vi "AOL Z Cal-Ctrl visibility.vi"(8 "error in (no error)":errorcluster, 11 "State":T1=enum."Select cal mode") -> (0 "error out":errorcluster)   [LabVIEW 2020]
uses:
  Typedefs/AOL Z cal wizard states.ctl
  Globals/gl_Calibration globals.vi
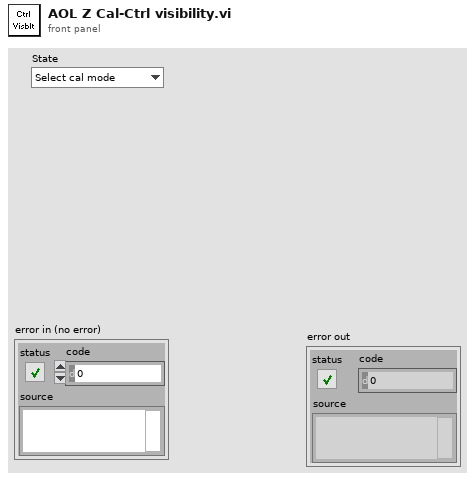
[diagram p1: front panel]
types:
  T1 = typedef "AOL Z cal wizard states.ctl" = enum16{"Idle", "Select cal mode", "Select cal points", "Select channel", "Start calibration"}
  T2 = enum8{"Enabled", "Disabled", "Disabled and Grayed Out"}
  T3 = typedef "Pre-AOL Z wizard refs.ctl" = cluster{"VI's reference":refnum<vi>, "Calibration Mode":refnum<vi>, "Cal points":refnum<vi>, "Channel Selector":refnum<vi>, "Message":refnum<vi>, "Back":refnum<vi>, "Next":refnum<vi>, "Power meter AI":refnum<vi>, "2D Picture":refnum<vi>, "Note":refnum<vi>}
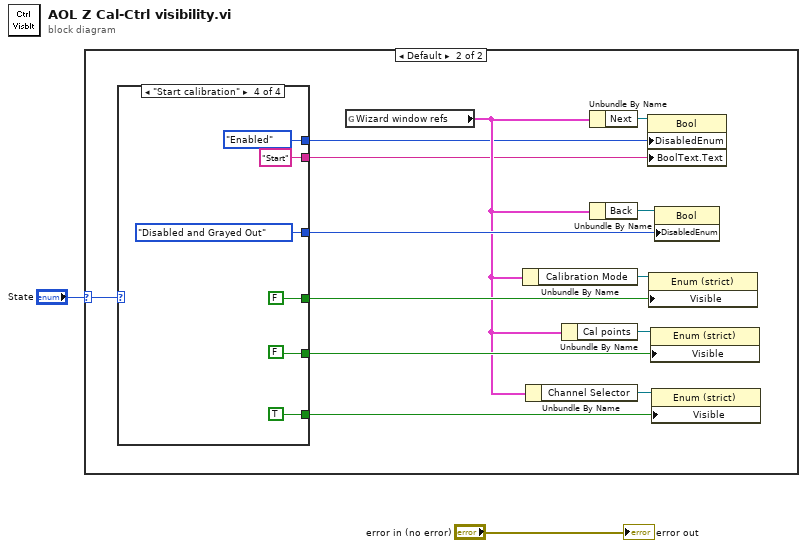
[diagram p0: block diagram]
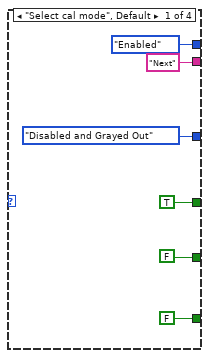
[diagram p3: hidden frame]
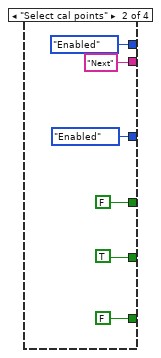
[diagram p4: hidden frame]
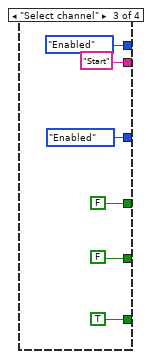
[diagram p5: hidden frame]
diagram:
  n1 = case shown="Default" "State" {
    selector: "State" -> [_ w12]
    frame "Idle" {
    }
    frame Default {
      n2 = case shown="\"Start calibration\"" w12 {
        tunnel: [TRUE FALSE FALSE FALSE] -> w11
        tunnel: [FALSE TRUE FALSE FALSE] -> w10
        tunnel: [FALSE FALSE TRUE TRUE] -> w9
        tunnel: [T2."Disabled and Grayed Out" ("Disabled") T2."Enabled" ("Disabled") T2."Enabled" ("Disabled") T2."Disabled and Grayed Out" ("Disabled")] -> w7
        tunnel: [T2."Enabled" ("Disabled") T2."Enabled" ("Disabled") T2."Enabled" ("Disabled") T2."Enabled" ("Disabled")] -> w4
        tunnel: ["Next" ("Boolean Text.Text") "Next" ("Boolean Text.Text") "Start" ("Boolean Text.Text") "Start" ("Boolean Text.Text")] -> w3
        frame "Select cal mode", Default {
        }
        frame "Select cal points" {
        }
        frame "Select channel" {
        }
        frame "Start calibration" {
        }
      }
      n3 = global read "gl_Calibration globals.vi" "Wizard window refs"() -> (w5:T3)
      n4 = Unbundle By Name(w5) -> ("Calibration Mode"=w13:refnum<vi>)
      n5 = Unbundle By Name(w5) -> ("Channel Selector"=w15:refnum<vi>)
      n6 = Unbundle By Name(w5) -> ("Cal points"=w14:refnum<vi>)
      n7 = Unbundle By Name(w5) -> ("Next"=w6:refnum<vi>)
      n8 = Unbundle By Name(w5) -> ("Back"=w8:refnum<vi>)
      n9 = property on="Property Node" class="Bool"(reference=w6, "DisabledEnum"=w4, "BoolText.Text"=w3) -> ()  [unwired: 1 in, 2 out]
      n10 = property on="Property Node" class="Enum (strict)"(reference=w13, "Visible"=w11) -> ()  [unwired: 1 in, 2 out]
      n11 = property on="Property Node" class="Enum (strict)"(reference=w14, "Visible"=w10) -> ()  [unwired: 1 in, 2 out]
      n12 = property on="Property Node" class="Enum (strict)"(reference=w15, "Visible"=w9) -> ()  [unwired: 1 in, 2 out]
      n13 = property on="Property Node" class="Bool"(reference=w8, "DisabledEnum"=w7) -> ()  [unwired: 1 in, 2 out]
    }
  }
  "error out" <- "error in (no error)"
